vi "Write Staff mode.vi"(8 "error in (no error)":errorcluster, 9 "Password":string, 10 "Staff mode":bool, 11 "PS Control Actor in":refnum<class "PS Control Actor.lvclass">) -> (0 "error out":errorcluster, 3 "PS Control Actor out":refnum<class "PS Control Actor.lvclass">)   [LabVIEW 2024, in "PS Control Actor.lvlib" / "PS Control Actor.lvclass"]
uses:
  PS Control Actor.lvclass
  C:/Program Files/National Instruments/LabVIEW 2024/vi.lib/ActorFramework/Actor/Actor.lvclass
  PS Control Actor.lvclass/PS Control Actor.ctl
  <vilib>/ActorFramework/Actor/Actor.lvclass/Actor.ctl
  <vilib>/ActorFramework/Message Enqueuer/Message Enqueuer.lvclass/Message Enqueuer.ctl
  <vilib>/ActorFramework/Message Enqueuer/Enqueue.vi
  <vilib>/ActorFramework/Message Enqueuer/Init from Existing Queue.vi
  PS Control Actor Messages/Update Mode Menu Items Msg/Update Mode Menu Items Msg.lvclass
  C:/Program Files/National Instruments/LabVIEW 2024/vi.lib/ActorFramework/Message/Message.lvclass
  <userlib>/_OpenG.lib/md5/md5.llb/MD5 Message Digest (Binary String)__ogtk.vi
  <vilib>/ActorFramework/Message Priority Queue/Priority Enqueue.vi
  <vilib>/ActorFramework/Message Enqueuer/Message Enqueuer.lvclass
  <vilib>/ActorFramework/Actor/Actor.lvclass
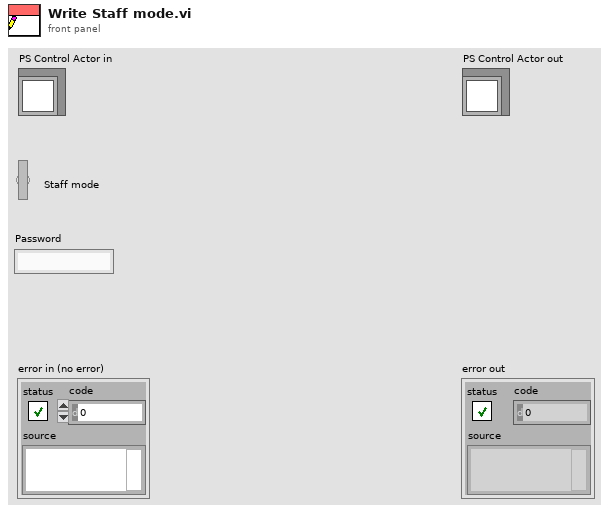
[diagram p1: front panel]
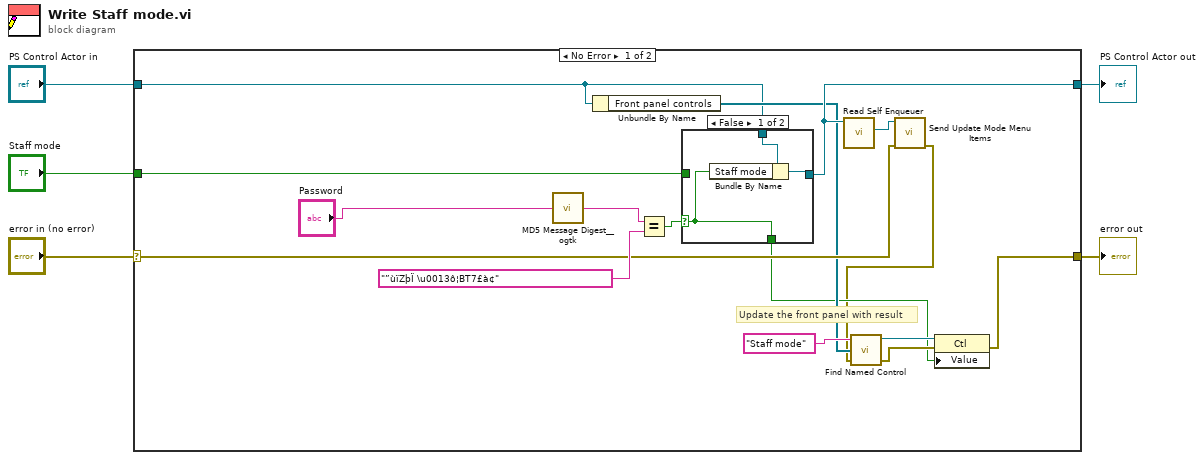
[diagram p0: block diagram]
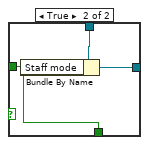
[diagram p2: hidden frame]
diagram:
  n1 = case shown="No Error" "error in (no error)" {
    selector: "error in (no error)" -> [w14 w29]
    tunnel: [w6 w29] -> w4
    tunnel: [w16 w28] -> w2
    tunnel: "PS Control Actor in" -> [w9 w28]
    tunnel: "Staff mode" -> [w21 _]
    frame No Error {
      # "Update the front panel with result"
      n2 = call-poly <userlib>:"MD5 Message Digest__ogtk.vi"("Message"="Password") -> ("MD5 Message Digest"=w20:string)
      n3 = Unbundle By Name(w9) -> ("Front panel controls"=w12:refnum<vi>[])
      n4 = Equal?(x=w20, y="”ùïZþÏ \u0013ô¦BT7£à¢" ("Password")) -> (x = y?=w17:bool)
      n5 = case shown="False" w17 {
        selector: w17 -> [w22 _]
        tunnel: w9 -> [w24 w27]
        tunnel: [w23 w26] -> w16
        tunnel: w21 -> [_ w25]
        tunnel: [w22 w25] -> w8
        frame False {
          n6 = Bundle By Name(cluster=w24, "Staff mode"=w22) -> (w23:refnum<class "PS Control Actor.lvclass">)
        }
        frame True {
          n7 = Bundle By Name(cluster=w27, "Staff mode"=w25) -> (w26:refnum<class "PS Control Actor.lvclass">)
        }
      }
      n8 = call <vilib>:"Read Self Enqueuer.vi"("Actor"=w16) -> ("Self Enqueuer"=w15:refnum<class "Message Enqueuer.lvclass">)  [unwired: 10 in]
      n9 = call "Send Update Mode Menu Items.vi"("error in (no error)"=w14, "Message Enqueuer"=w15) -> ("error out"=w7:errorcluster)  [unwired: 8 in, 1 out]
      n10 = call "Find Named Control.vi"("error in"=w7, "All Controls"=w12, "Control Name"="Staff mode") -> ("error out"=w10:errorcluster, "Ctl Refnum"=w11:refnum<vi>)  [unwired: 1 out]
      n11 = property class="Ctl"(reference=w11, error in=w10, "Value"=w8) -> (error out=w6:errorcluster)  [unwired: 1 out]
    }
    frame Error {
    }
  }
  "error out" <- w4
  "PS Control Actor out" <- w2
